vi "WinHostToFlexRIO.vi"() -> ()   [LabVIEW 2013]
uses:
  <vilib>/userdefined/High Color/nirio_resource_hc.ctl
  <vilib>/rvi/interface/common/niFpgaWaitOnOcc.vi
  <vilib>/FPGAPlugInAG/PXIe-7961R/niLvFpga_Open_PXIe-7961R.vi
  <vilib>/FPGAPlugInAG/PXIe-7961R/niLvFpga_Reset_PXIe-7961R.vi
  <vilib>/Utility/error.llb/Error Cluster From Error Code.vi
  <vilib>/rvi/errors/niLvFpgaAdjustHostInterfaceError.vi
  <vilib>/FPGAPlugInAG/PXIe-7961R/niLvFpga_Run_PXIe-7961R.vi
  <vilib>/FPGAPlugInAG/PXIe-7961R/niLvFpga_Close_PXIe-7961R.vi
  <vilib>/rvi/interface/nirviOpenFPGA/nirviOpenFPGA.xnode
  FPGA Bitfiles/PXIe-7961R_FlexRIOonlyResources_v1_1.lvbitx
  FlexRIOonlyResources.vi
  <vilib>/rvi/interface/nirviMethod/nirviMethod.xnode
  <vilib>/rvi/interface/nirviReadWriteControl/nirviReadWriteControl.xnode
  Control 1.ctl
  <vilib>/rvi/interface/nirviCloseFPGA/nirviCloseFPGA.xnode
  <vilib>/rvi/errors/niLvFpgaMergeErrorWithErrorCode.vi
  NiFpgaLv.dll
  <vilib>/FPGAPlugInAG/PXIe-7961R/niLvFpga_ConfigureFifo_PXIe-7961R.vi
  <vilib>/FPGAPlugInAG/PXIe-7961R/niLvFpga_StartFifo_PXIe-7961R.vi
panel:
  in  "Tab Control":T1(tab)
  out "Platform":enum8{"FlexRIO", "cRIO", "RSeries"}(ring)
  out "FPGAVIversion":u8[](array[numeric])
  out "InsertedIOModule ID":u32
  out "Expected IO Module ID":u32
  out "RIOAdapterCorrect":bool
  out "Fref":u32
  out "DevQualityStatus":u8
  out "DevTemp":i16
  out "DevProfile":u8
  out "DMATtoHOSTFrameType":u8[](array[numeric])
  out "DMATtoHOSTNCh":u16[](array[numeric])
  out "DMATtoHOSTSampleSize":u8[](array[numeric])
  out "DMATtoHOSTBlockNWords":u16[](array[numeric])
  out "error out":errorcluster
  out "SGNo":u8
  out "DMATtoHOSTOverflows":u16
  in  "DO0":bool
  in  "DO1":bool
  in  "DO2":bool
  in  "DO3":bool
  in  "DO4":bool
  in  "DO5":bool
  in  "DO6":bool
  in  "DO7":bool
  in  "DO8":bool
  in  "DO9":bool
  in  "DO10":bool
  in  "DO11":bool
  in  "DO12":bool
  in  "DO13":bool
  in  "DO14":bool
  in  "DO15":bool
  in  "DO16":bool
  in  "DO17":bool
  in  "DO18":bool
  in  "DO19":bool
  in  "DO20":bool
  in  "DO21":bool
  in  "DO22":bool
  in  "DO23":bool
  in  "DO24":bool
  in  "DO25":bool
  in  "DO26":bool
  in  "DO27":bool
  in  "DO28":bool
  in  "DO29":bool
  in  "DO30":bool
  in  "DO31":bool
  in  "DO32":bool
  in  "DO33":bool
  in  "DO34":bool
  in  "DO35":bool
  in  "DO36":bool
  in  "DO37":bool
  in  "DO38":bool
  in  "DO40":bool
  in  "DO39":bool
  in  "DO41":bool
  in  "DO42":bool
  in  "DO43":bool
  in  "DO44":bool
  in  "DO45":bool
  in  "DO46":bool
  in  "DO47":bool
  in  "DO48":bool
  in  "DO49":bool
  in  "DO50":bool
  in  "DO51":bool
  in  "DO52":bool
  in  "DO53":bool
  in  "auxAO0":i32
  in  "auxAO1":i32
  in  "auxAO2":i32
  in  "auxAO3":i32
  in  "auxAO4":i32
  in  "auxAO5":i32
  in  "auxAO6":i32
  in  "auxAO7":i32
  in  "auxAO8":i32
  in  "auxAO9":i32
  in  "auxAO10":i32
  in  "auxAO11":i32
  in  "auxAO12":i32
  in  "auxAO13":i32
  in  "auxAO14":i32
  in  "auxAO15":i32
  in  "DAQStartStop":bool
  in  "DebugMode":bool
  in  "AOEnable0":bool
  in  "SGUpdateRate0":u32=10000000
  in  "SGPhase0":u32
  in  "SGFreq0":u32
  in  "AO0":i16
  in  "DMATtoHOSTEnable0":bool
  in  "SamplingRate0":u32=10000
  in  "stop":bool
  in  "SGSignalType0":enum16{"DC", "Sine", "Square", "Triangle"}(ring)
  in  "SGAmp0":u16
  in  "AOEnable1":bool
  in  "SGUpdateRate1":u32
  in  "SGPhase1":u32
  in  "SGFreq1":u32
  in  "AO1":i32
  in  "SGAmp1":u16
  in  "SGSignalType1":enum16{"DC", "Sine", "Square", "Triangle"}(ring)
  in  "FlexRIO Device":T2
  in  "auxDO9":bool
  in  "auxDO10":bool
  in  "auxDO11":bool
  in  "auxDO14":bool
  in  "auxDO13":bool
  in  "auxDO12":bool
  in  "auxDO15":bool
  in  "auxDO5":bool
  in  "auxDO4":bool
  in  "auxDO3":bool
  in  "auxDO2":bool
  in  "auxDO1":bool
  in  "auxDO0":bool
  in  "auxDO6":bool
  in  "auxDO8":bool
  in  "auxDO7":bool
  out "auxAI0":i32
  out "auxAI1":i32
  out "auxAI2":i32
  out "auxAI3":i32
  out "auxAI4":i32
  out "auxAI5":i32
  out "auxAI6":i32
  out "auxAI7":i32
  out "auxAI8":i32
  out "auxAI9 2":i32
  out "auxAI10":i32
  out "auxAI11":i32
  out "auxAI12":i32
  out "auxAI13":i32
  out "auxAI14":i32
  out "auxAI15":i32
  out "auxDI11":bool
  out "auxDI12":bool
  out "auxDI13":bool
  out "auxDI14":bool
  out "DI21":bool
  out "DI22":bool
  out "DI23":bool
  out "DI24":bool
  out "DI29":bool
  out "DI30":bool
  out "auxDI5":bool
  out "auxDI4":bool
  out "auxDI3":bool
  out "auxDI2":bool
  out "auxDI1":bool
  out "auxDI0":bool
  out "auxDI6":bool
  out "auxDI7":bool
  out "auxDI8":bool
  out "auxDI9":bool
  out "auxDI10":bool
  out "auxDI15":bool
  out "DI0":bool
  out "DI1":bool
  out "DI2":bool
  out "DI3":bool
  out "DI4":bool
  out "DI5":bool
  out "DI6":bool
  out "DI7":bool
  out "DI8":bool
  out "DI9":bool
  out "DI10":bool
  out "DI11":bool
  out "DI12":bool
  out "DI13":bool
  out "DI14":bool
  out "DI15":bool
  out "DI16":bool
  out "DI17":bool
  out "DI18":bool
  out "DI19":bool
  out "DI20":bool
  out "DI25":bool
  out "DI26":bool
  out "DI27":bool
  out "DI28":bool
  out "DI31":bool
  out "DI32":bool
  out "DI33":bool
  out "DI34":bool
  out "DI35":bool
  out "DI36":bool
  out "DI37":bool
  out "DI38":bool
  out "DI39":bool
  out "DI40":bool
  out "DI41":bool
  out "DI42":bool
  out "DI43":bool
  out "DI44":bool
  out "DI45":bool
  out "DI46":bool
  out "DI47":bool
  out "DI48":bool
  out "DI49":bool
  out "DI50":bool
  out "DI51":bool
  out "DI52":bool
  out "DI53":bool
  # "Digital outputs"
  # "Signal generators"
  # "Auxiliar digital outputs"
  # "Auxiliar analog outputs"
  # "Digital outputs"
  # "Auxiliar analog inputs"
  # "Auxiliar digital inputs"
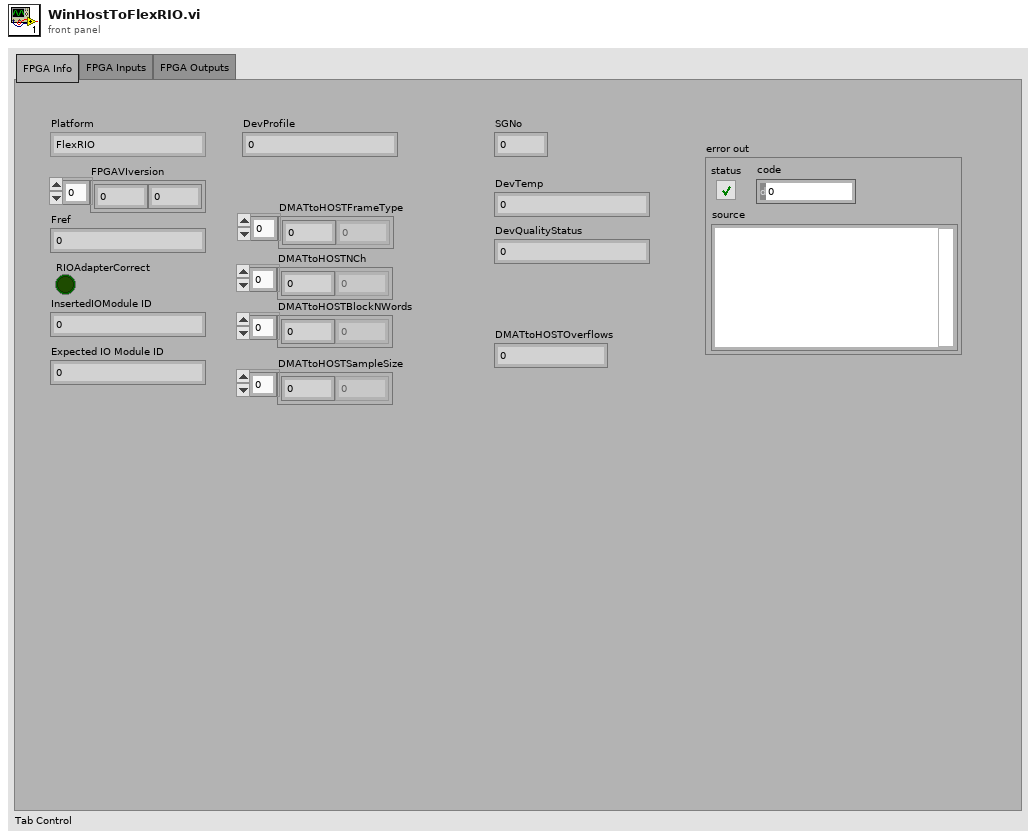
[diagram p1: front panel]
types:
  T1 = enum32{"FPGA Info", "FPGA Inputs", "FPGA Outputs"}
  T2 = typedef "nirio_resource_hc.ctl" = tag
  T3 = enum16{"DAQ-CPU", "IMAQ-CPU", "DAQ-GPU", "IMAQ-GPU"}
  T4 = typedef "Control 1.ctl" = u16
  T5 = cluster{"Timeout":u8, "Timeout":T4, "Timeout":u8, "Timeout":u16}
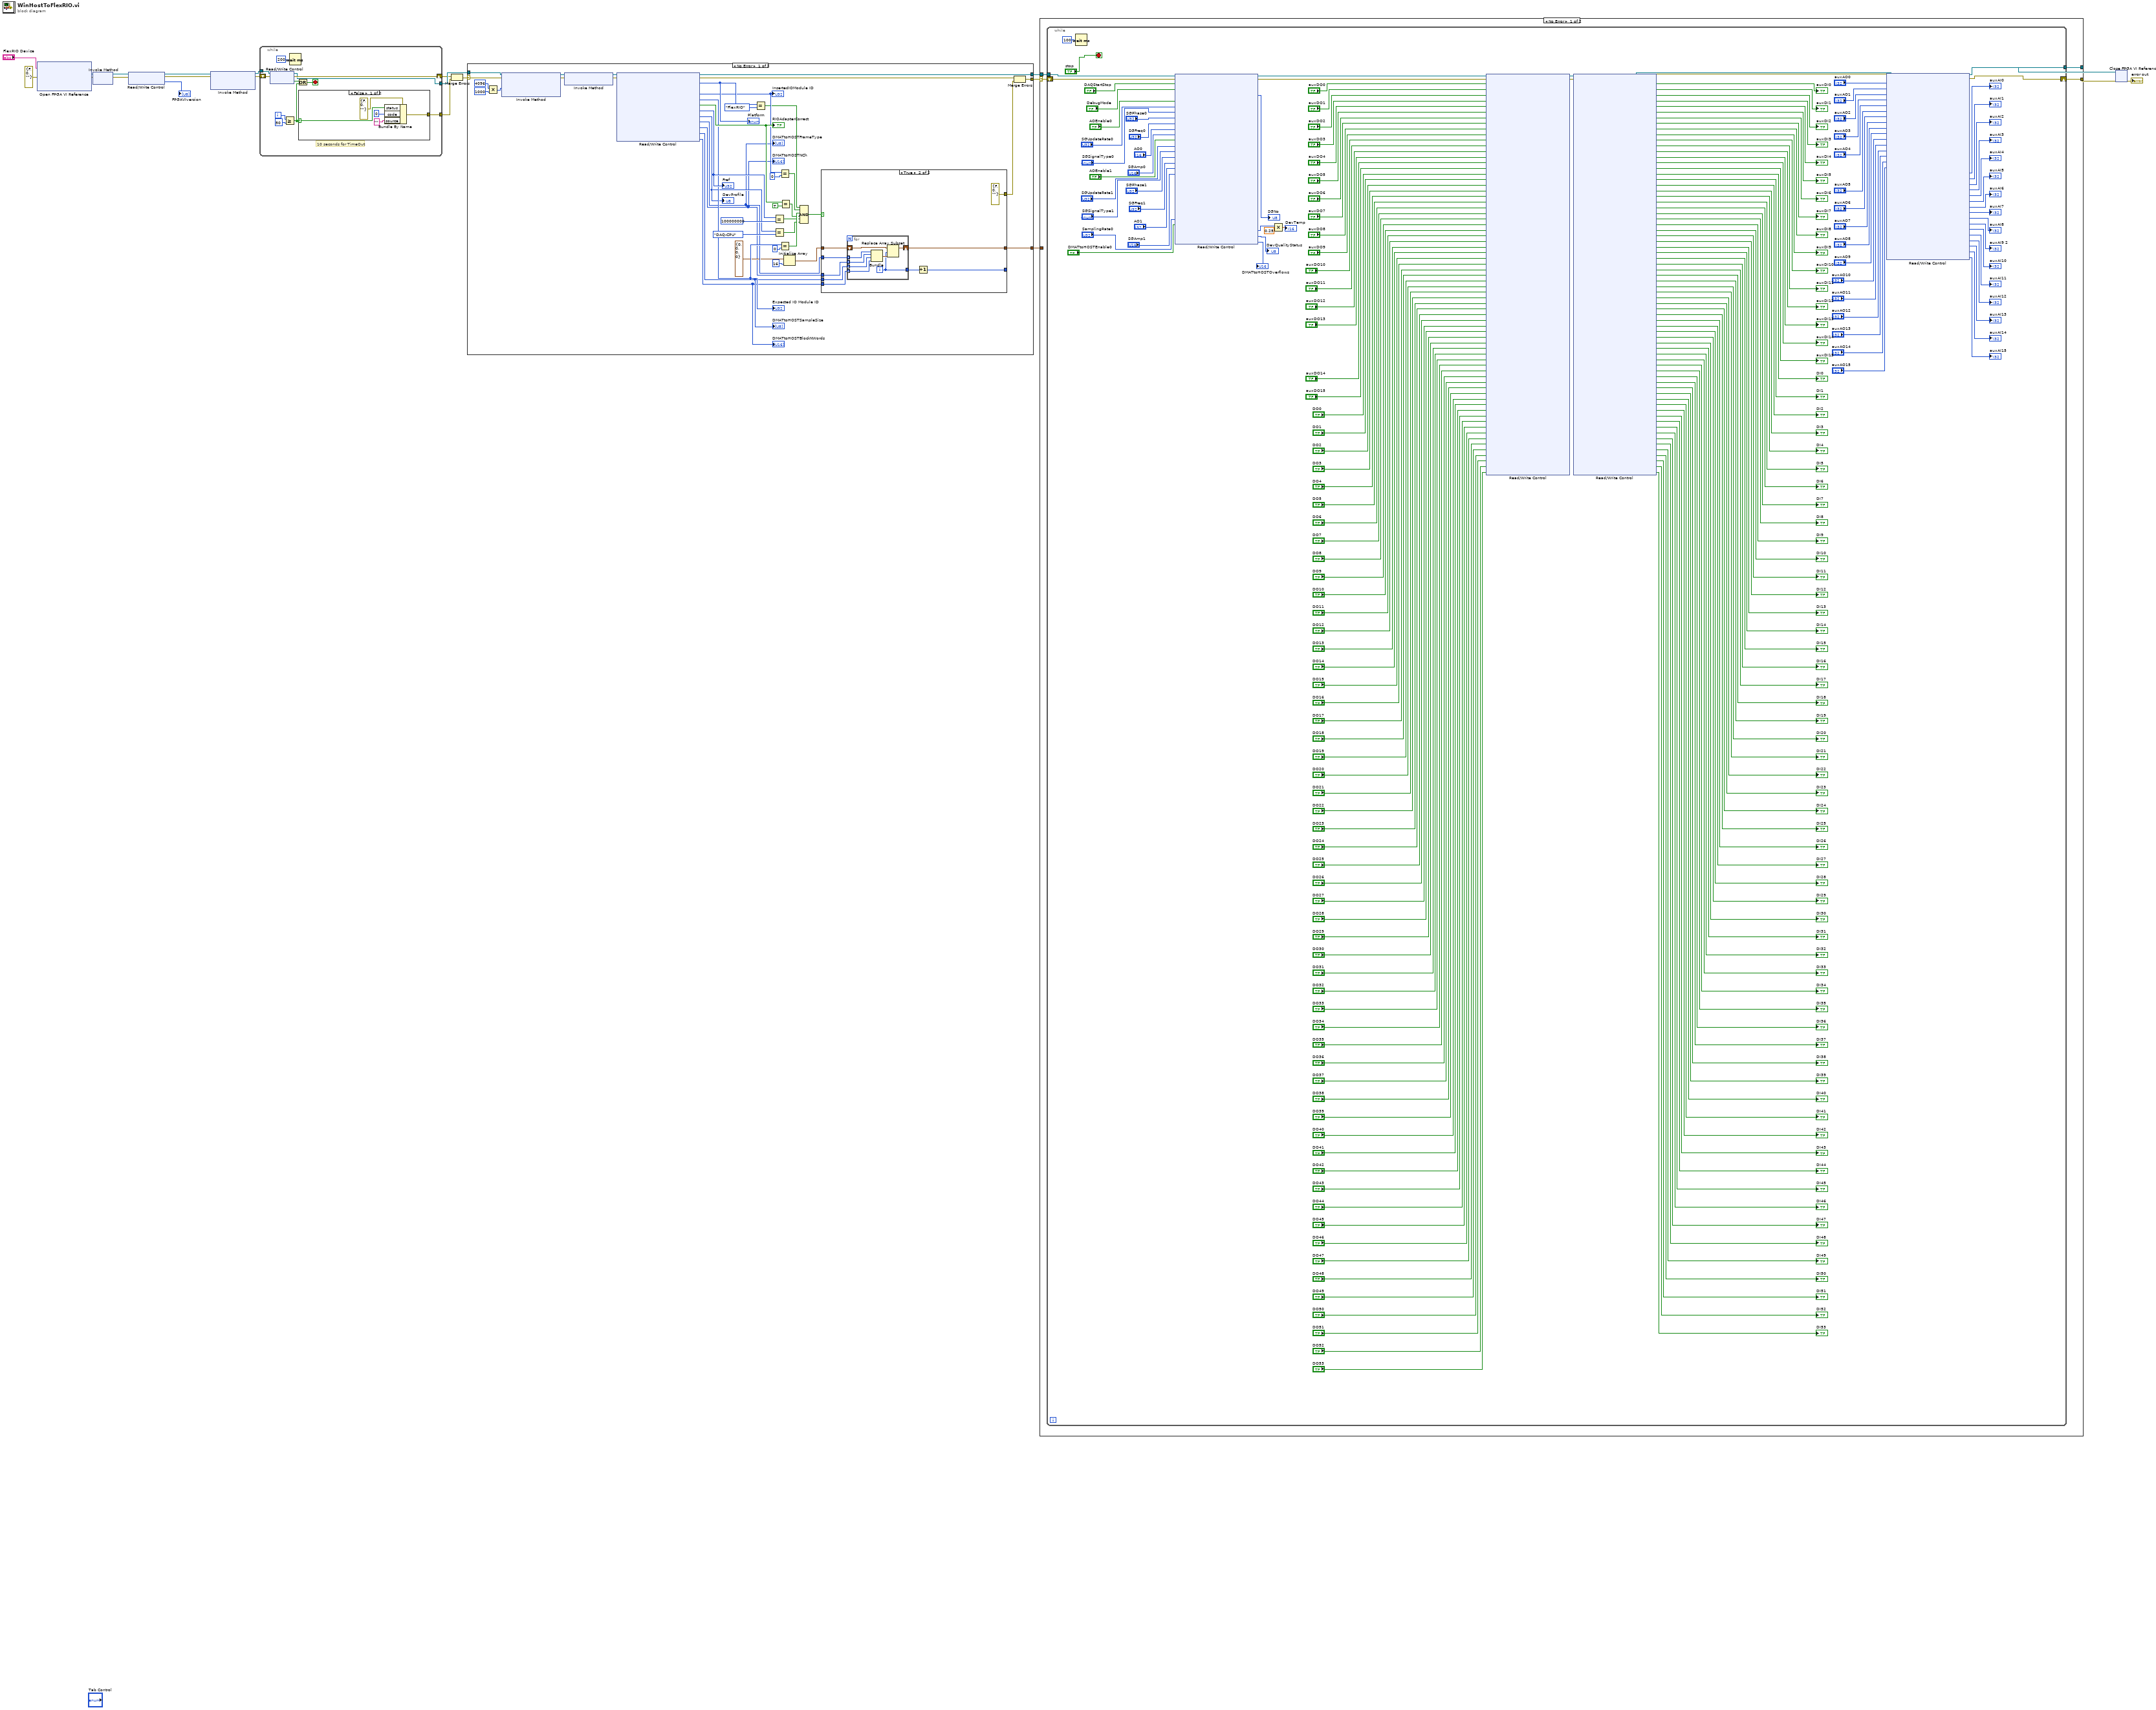
[diagram p0: block diagram]
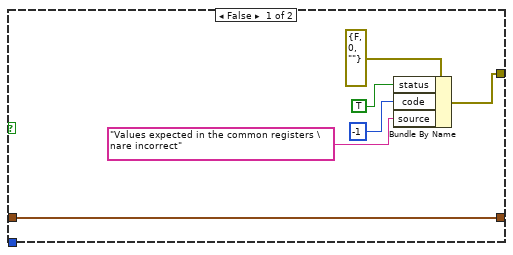
[diagram p3: hidden frame]
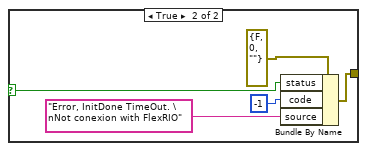
[diagram p5: hidden frame]
diagram:
  n1 = xnode "Open FPGA VI Reference"("error in"=errorcluster {"status"=FALSE, "code"=0, "source"=""}, "resource name"="FlexRIO Device") -> ("FPGA VI Reference Out"=w20:refnum<k20>, "error out"=w21:errorcluster)
  n2 = xnode "Invoke Method"("FPGA VI Reference In"=w20, "error in"=w21) -> ("FPGA VI Reference Out"=w1:refnum<k20>, "error out"=w2:errorcluster)
  n3 = xnode "Read/Write Control"("FPGA VI Reference In"=w1, "error in"=w2) -> ("FPGA VI Reference Out"=w4:refnum<k20>, "error out"=w3:errorcluster, "FPGAVIversion"=→"FPGAVIversion":u8[])
  n4 = xnode "Invoke Method"("FPGA VI Reference In"=w4, "error in"=w3) -> ("FPGA VI Reference Out"=w18:refnum<k20>, "error out"=w17:errorcluster)  [unwired: 1 in]
  n5 = while {
    tunnel: w18 -> [w32]
    tunnel: [w29] -> w16
    shift-right: [w30] -> w14
    shift-left: w17 -> [w31]
    tunnel: [w22] -> w15
    i -> [w27]
    stop <- w24 stop-if-true
    # "10 seconds for TimeOut"
    n6 = xnode "Read/Write Control"("FPGA VI Reference In"=w32, "error in"=w31) -> ("FPGA VI Reference Out"=w29:refnum<k20>, "error out"=w30:errorcluster, "InitDone"=w25:bool)
    n7 = Greater Or Equal?(x=w27, y=50) -> (x >= y?=w23:bool)
    n8 = Wait (ms)(milliseconds to wait=u32 200) -> ()  [unwired: 1 out]
    n9 = Or(x=w25, y=w23) -> (x .or. y?=w24:bool)
    n10 = case shown="False" w23 {
      selector: w23 -> [w34 w39]
      tunnel: [w33 w38] -> w22
      frame False {
        n11 = Bundle By Name(cluster=errorcluster {"status"=FALSE, "code"=0, "source"=""} ("error constant"), "status"=w34, "code"=0, "source"="") -> (w33:errorcluster)
      }
      frame True {
        n12 = Bundle By Name(cluster=errorcluster {"status"=FALSE, "code"=0, "source"=""} ("error constant"), "status"=w39, "code"=-1, "source"="Error, InitDone TimeOut. \nNot conexion with FlexRIO") -> (w38:errorcluster)
      }
    }
  }
  n13 = Merge Errors(w14, w15) -> (w13:errorcluster)
  n14 = case shown="No Error" w13 {
    selector: w13 -> [w76 w107]
    tunnel: w16 -> [w77 w106]
    tunnel: [w73 w106] -> w10
    tunnel: [w46 w107] -> w11
    tunnel: [w44 _] -> w7
    frame No Error {
      n15 = Multiply(x=u32 4096 ("Requested Depth"), y=u32 1000) -> (x*y=w78:u32)
      n16 = xnode "Invoke Method"("FPGA VI Reference In"=w77, "error in"=w76, "Requested Depth"=w78) -> ("FPGA VI Reference Out"=w82:refnum<k20>, "error out"=w81:errorcluster)  [unwired: 1 out]
      n17 = xnode "Invoke Method"("FPGA VI Reference In"=w82, "error in"=w81) -> ("FPGA VI Reference Out"=w74:refnum<k20>, "error out"=w75:errorcluster)
      n18 = xnode "Read/Write Control"("FPGA VI Reference In"=w74, "error in"=w75) -> ("FPGA VI Reference Out"=w73:refnum<k20>, "error out"=w47:errorcluster, "Platform"=w72:enum8{"FlexRIO", "cRIO", "RSeries"}, "InsertedIOModule ID"=w66:u32, "Expected IO Module ID"=w64:u32, "RIOAdapterCorrect"=w68:bool, "Fref"=w70:u32, "DevProfile"=w62:u8, "DMATtoHOSTFrameType"=w58:u8[], "DMATtoHOSTNCh"=w43:T4[], "DMATtoHOSTSampleSize"=w60:u8[], "DMATtoHOSTBlockNWords"=w59:u16[])  [unwired: 1 out]
      "Platform" <- w72
      "InsertedIOModule ID" <- w66
      "Expected IO Module ID" <- w64
      "RIOAdapterCorrect" <- w68
      "Fref" <- w70
      "DevProfile" <- w62
      "DMATtoHOSTFrameType" <- w58
      "DMATtoHOSTNCh" <- w43
      "DMATtoHOSTSampleSize" <- w60
      "DMATtoHOSTBlockNWords" <- w59
      n19 = Equal?(x=w72, y=enum16{"FlexRIO", "cRIO", "R-Series"}."FlexRIO") -> (x = y?=w56:bool)
      n20 = Equal?(x=w70, y=u32 100000000) -> (x = y?=w52:bool)
      n21 = Equal?(x=w62, y=T3."DAQ-CPU") -> (x = y?=w51:bool)
      n22 = Equal?(x=w66, y=u32 0) -> (x = y?=w55:bool)
      n23 = Equal?(x=w64, y=u32 0) -> (x = y?=w54:bool)
      n24 = Equal?(x=w68, y=TRUE) -> (x = y?=w53:bool)
      n25 = Initialize Array(cluster{u8, u16, u8, u16} {0, 0, 0, 0}, 16 ("dimension size")) -> (w48:cluster{u8, u16, u8, u16}[])
      n26 = Compound Arithmetic op=AND(w56, w55, w54, w53, w52, w51) -> (w57:bool)
      n27 = case shown="True" w57 {
        tunnel: w43 -> [_ w97]
        tunnel: w60 -> [_ w96]
        tunnel: w59 -> [_ w95]
        tunnel: w58 -> [_ w94]
        tunnel: w48 -> [w83 w93]
        tunnel: [w83 w92] -> w44
        tunnel: [w84 errorcluster {"status"=FALSE, "code"=0, "source"=""} ("error constant")] -> w45
        tunnel: [_ w89] -> _
        frame False {
          n28 = Bundle By Name(cluster=errorcluster {"status"=FALSE, "code"=0, "source"=""} ("error constant"), "status"=TRUE, "code"=-1, "source"="Values expected in the common registers \nare incorrect") -> (w84:errorcluster)
        }
        frame True {
          n29 = for {
            tunnel: w97 -> [w103] mode=indexing
            tunnel: w96 -> [w102] mode=indexing
            tunnel: w95 -> [w101] mode=indexing
            tunnel: w94 -> [w104] mode=indexing
            shift-right: [w99] -> w92
            shift-left: w93 -> [w105]
            tunnel: [w98] -> w90
            i -> [w98]
            n30 = Bundle("Timeout"=w104, "Timeout"=w103, "Timeout"=w102, "Timeout"=w101) -> (w100:T5)  [unwired: 1 in]
            n31 = Replace Array Subset(array=w105, new element=w100, index=w98) -> (w99:cluster{u8, u16, u8, u16}[])
          }
          n32 = Increment(x=w90) -> (x+1=w89:i32)
        }
      }
      n33 = Merge Errors(w47, w45) -> (w46:errorcluster)
    }
    frame Error {
    }
  }
  n34 = case shown="No Error" w11 {
    selector: w11 -> [w109 w321]
    tunnel: w10 -> [w110 w320]
    tunnel: [w108 w320] -> w9
    tunnel: [w111 w321] -> w8
    tunnel: w7 -> [_ _]
    frame No Error {
      n35 = while {
        shift-right: [w119] -> w111
        shift-left: w109 -> [w318]
        tunnel: w110 -> [w319]
        tunnel: [w120] -> w108
        stop <- "stop" stop-if-true
        n36 = Wait (ms)(milliseconds to wait=u32 100) -> ()  [unwired: 1 out]
        n37 = xnode "Read/Write Control"("FPGA VI Reference In"=w319, "error in"=w318, "DAQStartStop"="DAQStartStop", "DebugMode"="DebugMode", "AOEnable0"="AOEnable0", "SGUpdateRate0"="SGUpdateRate0", "SGSignalType0"="SGSignalType0", "SGPhase0"="SGPhase0", "SGFreq0"="SGFreq0", "AO0"="AO0", "SGAmp0"="SGAmp0", "AOEnable1"="AOEnable1", "SGUpdateRate1"="SGUpdateRate1", "SGSignalType1"="SGSignalType1", "SGPhase1"="SGPhase1", "SGFreq1"="SGFreq1", "AO1"="AO1", "SGAmp1"="SGAmp1", "DMATtoHOSTSamplingRate0"="SamplingRate0", "DMATtoHOSTEnable0"="DMATtoHOSTEnable0") -> ("FPGA VI Reference Out"=w297:refnum<k20>, "error out"=w296:errorcluster, "SGNo"=→"SGNo":u8, "DevTemp"=w115:i16, "DevQualityStatus"=→"DevQualityStatus":u8, "DMATtoHOSTOverflows"=→"DMATtoHOSTOverflows":u16)  [unwired: 7 out]
        n38 = Multiply(x=w115, y=sgl 0.25) -> (x*y=→"DevTemp":sgl)
        n39 = xnode "Read/Write Control"("FPGA VI Reference In"=w297, "error in"=w296, "auxDO0"="auxDO0", "auxDO1"="auxDO1", "auxDO2"="auxDO2", "auxDO3"="auxDO3", "auxDO4"="auxDO4", "auxDO5"="auxDO5", "auxDO6"="auxDO6", "auxDO7"="auxDO7", "auxDO8"="auxDO8", "auxDO9"="auxDO9", "auxDO10"="auxDO10", "auxDO11"="auxDO11", "auxDO12"="auxDO12", "auxDO13"="auxDO13", "auxDO14"="auxDO14", "auxDO15"="auxDO15", "DO0"="DO0", "DO1"="DO1", "DO2"="DO2", "DO3"="DO3", "DO4"="DO4", "DO5"="DO5", "DO6"="DO6", "DO7"="DO7", "DO8"="DO8", "DO9"="DO9", "DO10"="DO10", "DO11"="DO11", "DO12"="DO12", "DO13"="DO13", "DO14"="DO14", "DO15"="DO15", "DO16"="DO16", "DO17"="DO17", "DO18"="DO18", "DO19"="DO19", "DO20"="DO20", "DO21"="DO21", "DO22"="DO22", "DO23"="DO23", "DO24"="DO24", "DO25"="DO25", "DO26"="DO26", "DO27"="DO27", "DO28"="DO28", "DO29"="DO29", "DO30"="DO30", "DO31"="DO31", "DO32"="DO32", "DO33"="DO33", "DO34"="DO34", "DO35"="DO35", "DO36"="DO36", "DO37"="DO37", "DO38"="DO38", "DO39"="DO39", "DO40"="DO40", "DO41"="DO41", "DO42"="DO42", "DO43"="DO43", "DO44"="DO44", "DO45"="DO45", "DO46"="DO46", "DO47"="DO47", "DO48"="DO48", "DO49"="DO49", "DO50"="DO50", "DO51"="DO51", "DO52"="DO52", "DO53"="DO53") -> ("FPGA VI Reference Out"=w224:refnum<k20>, "error out"=w223:errorcluster)
        n40 = xnode "Read/Write Control"("FPGA VI Reference In"=w224, "error in"=w223) -> ("FPGA VI Reference Out"=w154:refnum<k20>, "error out"=w153:errorcluster, "auxDI0"=→"auxDI0":bool, "auxDI1"=→"auxDI1":bool, "auxDI2"=→"auxDI2":bool, "auxDI3"=→"auxDI3":bool, "auxDI4"=→"auxDI4":bool, "auxDI5"=→"auxDI5":bool, "auxDI6"=→"auxDI6":bool, "auxDI7"=→"auxDI7":bool, "auxDI8"=→"auxDI8":bool, "auxDI9"=→"auxDI9":bool, "auxDI10"=→"auxDI10":bool, "auxDI11"=→"auxDI11":bool, "auxDI12"=→"auxDI12":bool, "auxDI13"=→"auxDI13":bool, "auxDI14"=→"auxDI14":bool, "auxDI15"=→"auxDI15":bool, "DI0"=→"DI0":bool, "DI1"=→"DI1":bool, "DI2"=→"DI2":bool, "DI3"=→"DI3":bool, "DI4"=→"DI4":bool, "DI5"=→"DI5":bool, "DI6"=→"DI6":bool, "DI7"=→"DI7":bool, "DI8"=→"DI8":bool, "DI9"=→"DI9":bool, "DI10"=→"DI10":bool, "DI11"=→"DI11":bool, "DI12"=→"DI12":bool, "DI13"=→"DI13":bool, "DI14"=→"DI14":bool, "DI15"=→"DI15":bool, "DI16"=→"DI16":bool, "DI17"=→"DI17":bool, "DI18"=→"DI18":bool, "DI19"=→"DI19":bool, "DI20"=→"DI20":bool, "DI21"=→"DI21":bool, "DI22"=→"DI22":bool, "DI23"=→"DI23":bool, "DI24"=→"DI24":bool, "DI25"=→"DI25":bool, "DI26"=→"DI26":bool, "DI27"=→"DI27":bool, "DI28"=→"DI28":bool, "DI29"=→"DI29":bool, "DI30"=→"DI30":bool, "DI31"=→"DI31":bool, "DI32"=→"DI32":bool, "DI33"=→"DI33":bool, "DI34"=→"DI34":bool, "DI35"=→"DI35":bool, "DI36"=→"DI36":bool, "DI37"=→"DI37":bool, "DI38"=→"DI38":bool, "DI39"=→"DI39":bool, "DI40"=→"DI40":bool, "DI41"=→"DI41":bool, "DI42"=→"DI42":bool, "DI43"=→"DI43":bool, "DI44"=→"DI44":bool, "DI45"=→"DI45":bool, "DI46"=→"DI46":bool, "DI47"=→"DI47":bool, "DI48"=→"DI48":bool, "DI49"=→"DI49":bool, "DI50"=→"DI50":bool, "DI51"=→"DI51":bool, "DI52"=→"DI52":bool, "DI53"=→"DI53":bool)
        n41 = xnode "Read/Write Control"("FPGA VI Reference In"=w154, "error in"=w153, "auxAO0"="auxAO0", "auxAO1"="auxAO1", "auxAO2"="auxAO2", "auxAO3"="auxAO3", "auxAO4"="auxAO4", "auxAO5"="auxAO5", "auxAO6"="auxAO6", "auxAO7"="auxAO7", "auxAO8"="auxAO8", "auxAO9"="auxAO9", "auxAO10"="auxAO10", "auxAO11"="auxAO11", "auxAO12"="auxAO12", "auxAO13"="auxAO13", "auxAO14"="auxAO14", "auxAO15"="auxAO15") -> ("FPGA VI Reference Out"=w120:refnum<k20>, "error out"=w119:errorcluster, "auxAI0"=→"auxAI0":i32, "auxAI1"=→"auxAI1":i32, "auxAI2"=→"auxAI2":i32, "auxAI3"=→"auxAI3":i32, "auxAI4"=→"auxAI4":i32, "auxAI5"=→"auxAI5":i32, "auxAI6"=→"auxAI6":i32, "auxAI7"=→"auxAI7":i32, "auxAI8"=→"auxAI8":i32, "auxAI9"=→"auxAI9 2":i32, "auxAI10"=→"auxAI10":i32, "auxAI11"=→"auxAI11":i32, "auxAI12"=→"auxAI12":i32, "auxAI13"=→"auxAI13":i32, "auxAI14"=→"auxAI14":i32, "auxAI15"=→"auxAI15":i32)
      }
    }
    frame Error {
    }
  }
  n42 = xnode "Close FPGA VI Reference"("FPGA VI Reference In"=w9, "error in"=w8) -> ("error out"=→"error out":errorcluster)
